vi "Read gRPCid.vi"(8 "error in":errorcluster, 11 "ServiceBase in":refnum<class "ServiceBase.lvclass">) -> (0 "error out":errorcluster, 2 "gRPCid":T1, 3 "ServiceBase out":refnum<class "ServiceBase.lvclass">)   [LabVIEW 2024, in "gRPC-servicer.lvlib" / "ServiceBase.lvclass"]
uses:
  ServiceBase.lvclass
  gRPC lv Support/grpc-lvsupport/grpcId.ctl
  ServiceBase.lvclass/ServiceBase.ctl
  gRPC lv Support/grpc-lvsupport/grpc-lvsupport.lvlib
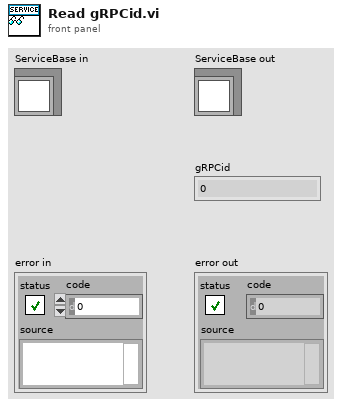
[diagram p1: front panel]
types:
  T1 = typedef "grpc-lvsupport.lvlib/grpcId.ctl" = u64
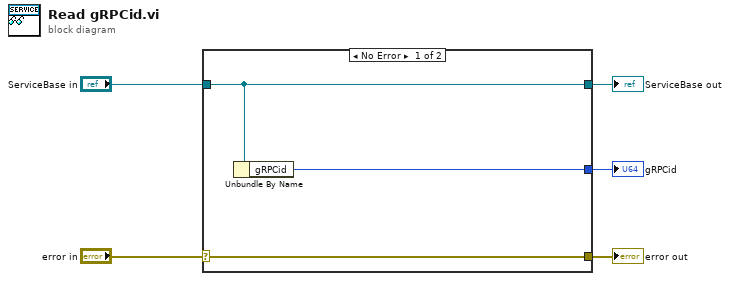
[diagram p0: block diagram]
diagram:
  n1 = case shown="No Error" "error in" {
    selector: "error in" -> [w8 w10]
    tunnel: [w8 w10] -> w4
    tunnel: [w7 w9] -> w2
    tunnel: "ServiceBase in" -> [w7 w9]
    tunnel: [w6 _] -> w1
    frame No Error {
      n2 = Unbundle By Name(w7) -> ("gRPCid"=w6:T1)
    }
    frame Error {
    }
  }
  "error out" <- w4
  "ServiceBase out" <- w2
  "gRPCid" <- w1
